vi "Teleop.vi"(10 "Match Info":T1={"Autonomous Elapsed Seconds"=0.0, "TeleOp Elapsed Seconds"=0.0, "Disabled Elapsed Seconds"=0.0, "Visited Autonomous"=FALSE, "Visited TeleOp"=FALSE, "Visited Disabled"=FALSE, "Autonomous Settings"={"Autonomous Style"=enum."Independent", "VI Refnum"=refnum}}, 11 "Call Context":T2) -> ()   [LabVIEW 2017]
doc: "This VI is called for each TeleOp packet received from the DS where the robot is not disabled. It is often used to read from the joysticks and update I/O or to update setpoints for timed control loops. It should complete and return within 20 milliseconds or it may miss DS packets."
uses:
  <vilib>/Rock Robotics/WPI/DriverStation/WPI_DriverStationDerivedRobotMode.ctl
  <vilib>/Rock Robotics/WPI/DriverStation/WPI_DriverStationMatch Info.ctl
  <vilib>/Rock Robotics/WPI/Solenoid/WPI_SolenoidValue.ctl
  <vilib>/Rock Robotics/WPI/Utilities/WPI_GetSetVariantRefNum.vi
  <vilib>/Rock Robotics/Network Tables/NT Read Boolean.vi
  <vilib>/Rock Robotics/Network Tables/NT Read Number.vi
  Robot Global Data.vi
  <vilib>/Rock Robotics/WPI/ThirdParty/Phoenix-LabVIEW/Motor Controller/Get/CTRE_Phoenix_MotorController_GetQuadratureData.vi
  <vilib>/Rock Robotics/WPI/Solenoid/WPI_SolenoidSetEnum.vi
panel:
  out "Sample Slider 0":dbl(slide) scale=0.0..5.0
  out "Sample Boolean 1":bool
  out "Sample Boolean 0":bool
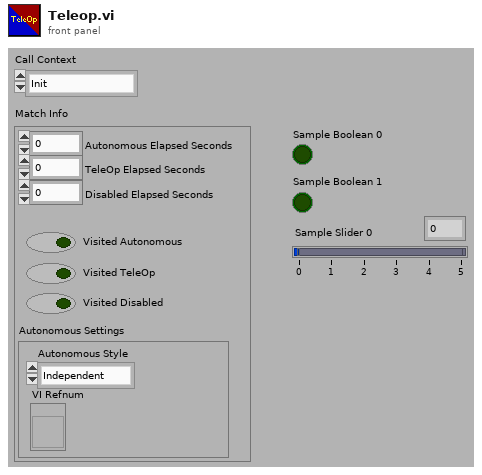
[diagram p1: front panel]
types:
  T1 = typedef "WPI_DriverStationMatch Info.ctl" = cluster{"Autonomous Elapsed Seconds":dbl, "TeleOp Elapsed Seconds":dbl, "Disabled Elapsed Seconds":dbl, "Visited Autonomous":bool, "Visited TeleOp":bool, "Visited Disabled":bool, "Autonomous Settings":cluster{"Autonomous Style":enum16{"Iterative", "Independent"}, "VI Refnum":refnum<vi>}}
  T2 = typedef "WPI_DriverStationDerivedRobotMode.ctl" = enum16{"Init", "Execute", "Stop"}
  T3 = typedef "WPI_SolenoidValue.ctl" = enum16{"Off", "On", "Forward", "Reverse"}
  T4 = typedef "WPI_JoystickDevRef.ctl" = cluster{"Device":T5}
  T5 = typedef "WPI_JoystickDeviceEnum.ctl" = enum16{"USB 0", "USB 1", "USB 2", "USB 3", "USB 4", "USB 5"}
  T6 = typedef "WPI_MotorControlDeviceRef.ctl" = cluster{"DeviceStatus":errorcluster, "Type":T7, "PWM":cluster{"PWM Channel":T8, "DeadBand":T9}, "CAN":cluster{"Device Number":u8, "SetOutput VI Ref":variant, "GetOutput VI Ref":variant, "Enable VI Ref":variant, "Disable VI Ref":variant, "Data":variant}, "Invert":bool, "DIO PWM":cluster{"PWM \"Enable\" Channel":T8, "DIOChannel":T10, "PWM Rate":dbl}}
  T7 = typedef "WPI_MotorControlType.ctl" = enum16{"PWM", "CAN", "DIO PWM"}
  T8 = typedef "FPGA_DIOPWMChannel.ctl" = enum8{"PWM 0", "PWM 1", "PWM 2", "PWM 3", "PWM 4", "PWM 5", "PWM 6", "PWM 7", "PWM 8", "PWM 9", "PWM MXP 0", "PWM MXP 1", "PWM MXP 2", "PWM MXP 3", "PWM MXP 4", "PWM MXP 5", "PWM MXP 6", "PWM MXP 7", "PWM MXP 8", "PWM MXP 9", "Invalid"}
  T9 = typedef "WPI_PWMDeadband.ctl" = cluster{"Name":string, "maxPositivePwm":i32, "minPositivePwm":i32, "centerPwm":i32, "maxNegativePwm":i32, "minNegativePwm":i32, "angularRange":u16}
  T10 = typedef "FPGA_DIOChannel.ctl" = enum8{"DIO 0", "DIO 1", "DIO 2", "DIO 3", "DIO 4", "DIO 5", "DIO 6", "DIO 7", "DIO 8", "DIO 9", "DIO MXP 0", "DIO MXP 1", "DIO MXP 2", "DIO MXP 3", "DIO MXP 4", "DIO MXP 5", "DIO MXP 6", "DIO MXP 7", "DIO MXP 8", "DIO MXP 9", "DIO MXP 10", "DIO MXP 11", "DIO MXP 12", "DIO MXP 13", "DIO MXP 14", "DIO MXP 15", "SPI Port CS1", "SPI Port CS2", "SPI Port CS3", "SPI Port MISO", "SPI Port MOSI", "Invalid"}
  T11 = typedef "WPI_SolenoidDevRef.ctl" = cluster{"DevStatus":errorcluster, "Pneumatics Control Module":u8, "Forward Solenoid Channel":T12, "Reverse Solenoid Channel":T12}
  T12 = typedef "WPI_SolenoidChannel.ctl" = enum8{"Solenoid 0", "Solenoid 1", "Solenoid 2", "Solenoid 3", "Solenoid 4", "Solenoid 5", "Solenoid 6", "Solenoid 7", "Invalid"}
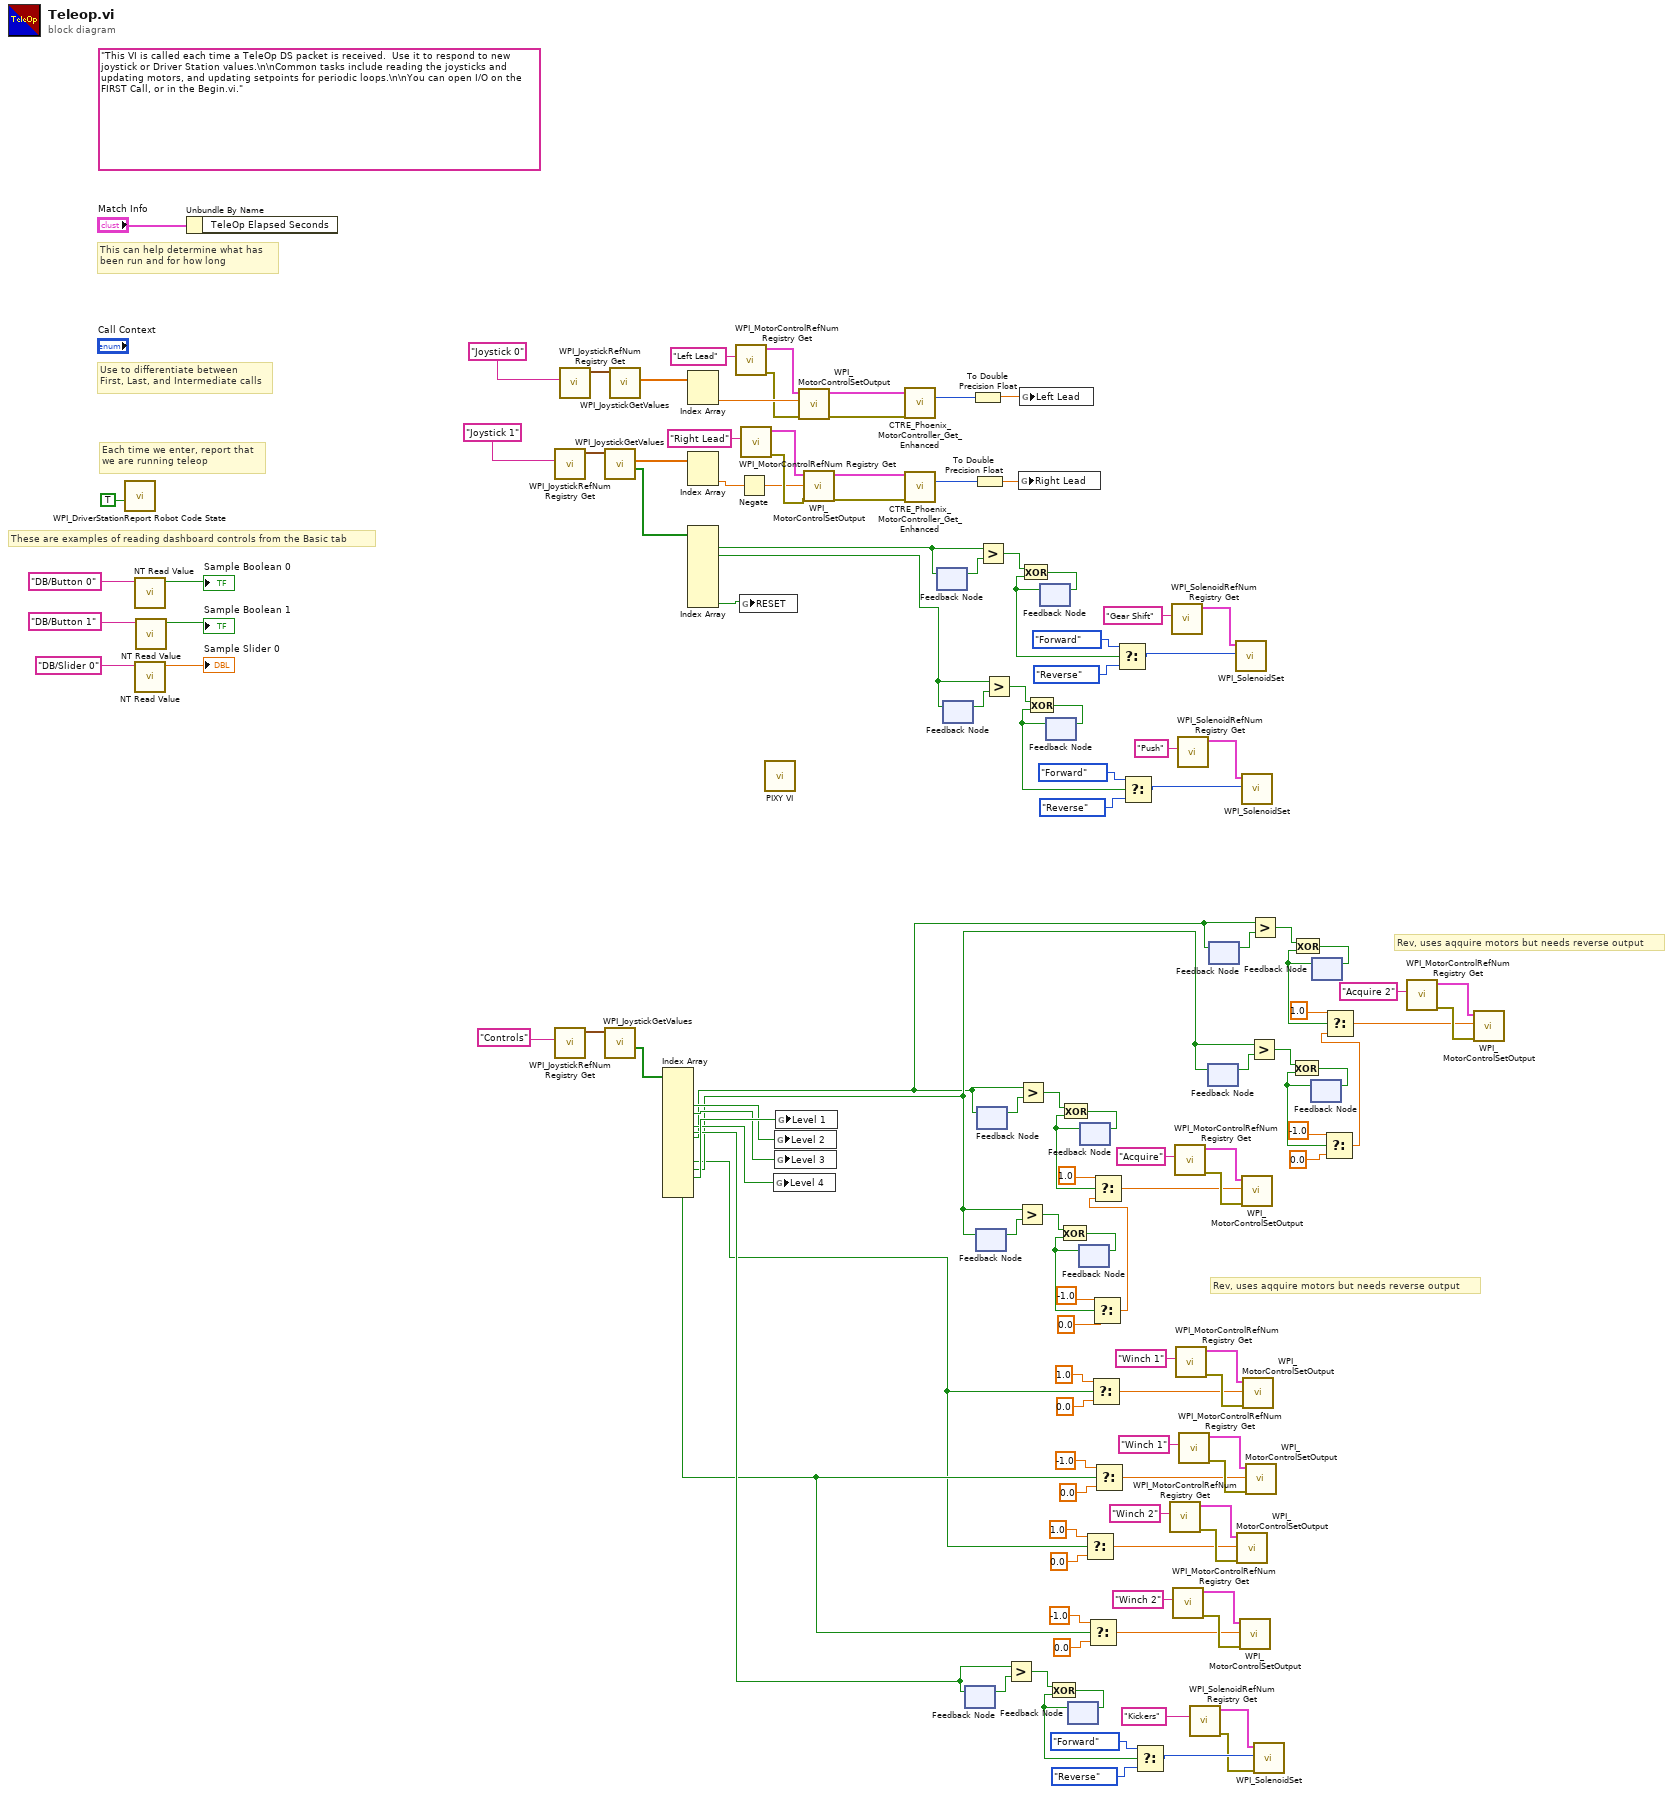
[diagram p0: block diagram]
diagram:
  (unwired) "This VI is called each time a TeleOp DS packet is received.  Use it to respond to new joystick or Driver Station values.\n\nCommon tasks include reading the joysticks and updating motors, and updating setpoints for periodic loops.\n\nYou can open I/O on the FIRST Call, or in the Begin.vi."
  # "Rev, uses aqquire motors but needs reverse output"
  # "Rev, uses aqquire motors but needs reverse output"
  # "These are examples of reading dashboard controls from the Basic tab"
  # "Each time we enter, report that\nwe are running teleop"
  # "Use to differentiate between\nFirst, Last, and Intermediate calls"
  # "This can help determine what has\nbeen run and for how long"
  n1 = call <vilib>:"WPI_DriverStationReport Robot Code State.vi"("TeleOp"=TRUE ("Autonomous")) -> ()  [unwired: 10 in, 1 out]
  n2 = call-poly <vilib>:"NT Read Value.vi"("Name"="DB/Button 0" ("refnum name")) -> ("Boolean"=→"Sample Boolean 0":bool)  [unwired: 9 in, 1 out]
  n3 = call-poly <vilib>:"NT Read Value.vi"("Name"="DB/Slider 0" ("refnum name")) -> ("Numeric"=→"Sample Slider 0":dbl)  [unwired: 9 in, 1 out]
  n4 = call-poly <vilib>:"NT Read Value.vi"("Name"="DB/Button 1" ("refnum name")) -> ("Boolean"=→"Sample Boolean 1":bool)  [unwired: 9 in, 1 out]
  n5 = Unbundle By Name("Match Info") -> ()  [unwired: 1 out]
  n6 = call <vilib>:"WPI_JoystickRefNum Registry Get.vi"("refnum name"="Joystick 1") -> ("JoystickDevRef"=w119:T4)  [unwired: 1 in, 9 out]
  n7 = call <vilib>:"WPI_JoystickRefNum Registry Get.vi"("refnum name"="Controls") -> ("JoystickDevRef"=w89:T4)  [unwired: 1 in, 9 out]
  n8 = call <vilib>:"WPI_JoystickRefNum Registry Get.vi"("refnum name"="Joystick 0") -> ("JoystickDevRef"=w129:T4)  [unwired: 1 in, 9 out]
  n9 = call <vilib>:"WPI_JoystickGetValues.vi"("JoystickDevRef"=w119) -> ("Buttons"=w112:bool[], "Axes"=w118:dbl[])  [unwired: 6 in, 3 out]
  n10 = call <vilib>:"WPI_JoystickGetValues.vi"("JoystickDevRef"=w89) -> ("Buttons"=w88:bool[])  [unwired: 6 in, 4 out]
  n11 = call <vilib>:"WPI_JoystickGetValues.vi"("JoystickDevRef"=w129) -> ("Axes"=w127:dbl[])  [unwired: 6 in, 4 out]
  n12 = Index Array(array=w88) -> (element #3=w36:bool, element #4=w38:bool, element #5=w37:bool, element #6=w35:bool, element #7=w16:bool, element #10=w1:bool, element #11=w17:bool, element #12=w39:bool, element #14=w2:bool)  [unwired: 14 in, 5 out]
  n13 = Index Array(array=w127) -> (element #1=w116:dbl)  [unwired: 2 in, 1 out]
  n14 = Index Array(array=w118) -> (element #2=w34:dbl)  [unwired: 2 in, 1 out]
  n15 = Index Array(array=w112) -> (element #1=w107:bool, element #2=w92:bool, element #8=w91:bool)  [unwired: 8 in, 5 out]
  n16 = call <vilib>:"WPI_MotorControlRefNum Registry Get.vi"("refnum name"="Left Lead") -> ("error out"=w78:errorcluster, "MotorControlDevRef"=w115:T6)  [unwired: 9 in]
  n17 = Negate(x=w34) -> (-x=w33:dbl)
  n18 = global write "Robot Global Data.vi" "RESET"(w91) -> ()
  n19 = call <vilib>:"WPI_MotorControlRefNum Registry Get.vi"("refnum name"="Right Lead") -> ("error out"=w79:errorcluster, "MotorControlDevRef"=w113:T6)  [unwired: 9 in]
  n20 = call "PIXY VI.vi"() -> ()  [unwired: 14 in, 6 out]
  n21 = global write "Robot Global Data.vi" "Level 4"(w37) -> ()
  n22 = global write "Robot Global Data.vi" "Level 2"(w36) -> ()
  n23 = global write "Robot Global Data.vi" "Level 3"(w38) -> ()
  n24 = global write "Robot Global Data.vi" "Level 1"(w39) -> ()
  n25 = call <vilib>:"WPI_MotorControlSetOutput.vi"("error in (no error)"=w78, "Output"=w116, "MotorControlDevRef"=w115) -> ("error out"=w63:errorcluster, "MotorControlDevRef"=w64:T6)  [unwired: 6 in, 1 out]
  n26 = call <vilib>:"WPI_MotorControlSetOutput.vi"("error in (no error)"=w79, "Output"=w33, "MotorControlDevRef"=w113) -> ("error out"=w59:errorcluster, "MotorControlDevRef"=w60:T6)  [unwired: 6 in, 1 out]
  n27 = call-poly <vilib>:"CTRE_Phoenix_MotorController_Get_Enhanced.vi"("PhoenixMotorControlDevRef"=w64, "error in"=w63) -> ("Quadrature Position"=w62:i32)  [unwired: 10 in, 3 out]
  n28 = call-poly <vilib>:"CTRE_Phoenix_MotorController_Get_Enhanced.vi"("PhoenixMotorControlDevRef"=w60, "error in"=w59) -> ("Quadrature Position"=w61:i32)  [unwired: 10 in, 3 out]
  n29 = feedback #1() -> (w108:bool)  [unwired: 1 in]
  n30 = feedback-in #1(w107) -> ()
  n31 = feedback #2() -> (w98:bool)  [unwired: 1 in]
  n32 = feedback-in #2(w92) -> ()
  n33 = feedback #3() -> (w45:bool)  [unwired: 1 in]
  n34 = feedback-in #3(w35) -> ()
  n35 = To Double Precision Float(number=w62) -> (double precision float=w58:dbl)
  n36 = To Double Precision Float(number=w61) -> (double precision float=w57:dbl)
  n37 = feedback #4() -> (w75:bool)  [unwired: 1 in]
  n38 = feedback-in #4(w17) -> ()
  n39 = feedback #5() -> (w85:bool)  [unwired: 1 in]
  n40 = feedback-in #5(w16) -> ()
  n41 = Greater?(x=w107, y=w108) -> (0:w111:bool)
  n42 = Greater?(x=w92, y=w98) -> (0:w101:bool)
  n43 = Greater?(x=w35, y=w45) -> (0:w46:bool)
  n44 = Greater?(x=w17, y=w75) -> (0:w77:bool)
  n45 = Greater?(x=w16, y=w85) -> (0:w87:bool)
  n46 = global write "Robot Global Data.vi" "Right Lead"(w57) -> ()
  n47 = global write "Robot Global Data.vi" "Left Lead"(w58) -> ()
  n48 = feedback #6() -> (w109:bool)  [unwired: 1 in]
  n49 = Exclusive Or(1:w109, 2:w111) -> (0:w110:bool)
  n50 = feedback-in #6(w110) -> ()
  n51 = feedback #7() -> (w99:bool)  [unwired: 1 in]
  n52 = Exclusive Or(1:w99, 2:w101) -> (0:w100:bool)
  n53 = feedback-in #7(w100) -> ()
  n54 = feedback #8() -> (w43:bool)  [unwired: 1 in]
  n55 = Exclusive Or(1:w43, 2:w46) -> (0:w44:bool)
  n56 = feedback-in #8(w44) -> ()
  n57 = feedback #9() -> (w74:bool)  [unwired: 1 in]
  n58 = Exclusive Or(1:w74, 2:w77) -> (0:w76:bool)
  n59 = feedback-in #9(w76) -> ()
  n60 = feedback #10() -> (w84:bool)  [unwired: 1 in]
  n61 = Exclusive Or(1:w84, 2:w87) -> (0:w86:bool)
  n62 = feedback-in #10(w86) -> ()
  n63 = Select(t=1.0, s=w1, f=0.0) -> (s? t:f=w9:dbl)
  n64 = Select(t=-1.0, s=w2, f=0.0) -> (s? t:f=w5:dbl)
  n65 = Select(t=1.0, s=w1, f=0.0) -> (s? t:f=w66:dbl)
  n66 = Select(t=-1.0, s=w74, f=0.0) -> (s? t:f=w42:dbl)
  n67 = Select(t=1.0, s=w84, f=w42) -> (s? t:f=w65:dbl)
  n68 = Select(t=-1.0, s=w2, f=0.0) -> (s? t:f=w53:dbl)
  n69 = Select(t=WPI_SolenoidValue."Forward" ("Value"), s=w109, f=WPI_SolenoidValue."Reverse" ("Value")) -> (s? t:f=w102:T3)
  n70 = Select(t=WPI_SolenoidValue."Forward" ("Value"), s=w99, f=WPI_SolenoidValue."Reverse" ("Value")) -> (s? t:f=w93:T3)
  n71 = Select(t=WPI_SolenoidValue."Forward" ("Value"), s=w43, f=WPI_SolenoidValue."Reverse" ("Value")) -> (s? t:f=w49:T3)
  n72 = call <vilib>:"WPI_MotorControlRefNum Registry Get.vi"("refnum name"="Winch 2") -> ("error out"=w10:errorcluster, "MotorControlDevRef"=w11:T6)  [unwired: 9 in]
  n73 = call <vilib>:"WPI_SolenoidRefNum Registry Get.vi"("refnum name"="Gear Shift") -> ("SolenoidDevRef"=w105:T11)  [unwired: 9 in, 1 out]
  n74 = call <vilib>:"WPI_MotorControlRefNum Registry Get.vi"("refnum name"="Winch 2") -> ("error out"=w6:errorcluster, "MotorControlDevRef"=w4:T6)  [unwired: 9 in]
  n75 = call <vilib>:"WPI_MotorControlRefNum Registry Get.vi"("refnum name"="Acquire") -> ("error out"=w80:errorcluster, "MotorControlDevRef"=w81:T6)  [unwired: 9 in]
  n76 = call <vilib>:"WPI_MotorControlRefNum Registry Get.vi"("refnum name"="Winch 1") -> ("error out"=w67:errorcluster, "MotorControlDevRef"=w68:T6)  [unwired: 9 in]
  n77 = call <vilib>:"WPI_SolenoidRefNum Registry Get.vi"("refnum name"="Push") -> ("SolenoidDevRef"=w96:T11)  [unwired: 9 in, 1 out]
  n78 = call <vilib>:"WPI_MotorControlRefNum Registry Get.vi"("refnum name"="Winch 1") -> ("error out"=w54:errorcluster, "MotorControlDevRef"=w52:T6)  [unwired: 9 in]
  n79 = call <vilib>:"WPI_SolenoidRefNum Registry Get.vi"("refnum name"="Kickers") -> ("error out"=w47:errorcluster, "SolenoidDevRef"=w48:T11)  [unwired: 9 in]
  n80 = feedback #11() -> (w22:bool)  [unwired: 1 in]
  n81 = feedback-in #11(w17) -> ()
  n82 = feedback #12() -> (w30:bool)  [unwired: 1 in]
  n83 = feedback-in #12(w16) -> ()
  n84 = call-poly <vilib>:"WPI_SolenoidSet.vi"("Value"=w102, "SolenoidDevRef"=w105) -> ()  [unwired: 8 in, 2 out]
  n85 = call <vilib>:"WPI_MotorControlSetOutput.vi"("error in (no error)"=w10, "Output"=w9, "MotorControlDevRef"=w11) -> ()  [unwired: 6 in, 3 out]
  n86 = call <vilib>:"WPI_MotorControlSetOutput.vi"("error in (no error)"=w6, "Output"=w5, "MotorControlDevRef"=w4) -> ()  [unwired: 6 in, 3 out]
  n87 = call-poly <vilib>:"WPI_SolenoidSet.vi"("Value"=w93, "SolenoidDevRef"=w96) -> ()  [unwired: 8 in, 2 out]
  n88 = call <vilib>:"WPI_MotorControlSetOutput.vi"("error in (no error)"=w80, "Output"=w65, "MotorControlDevRef"=w81) -> ()  [unwired: 6 in, 3 out]
  n89 = call <vilib>:"WPI_MotorControlSetOutput.vi"("error in (no error)"=w67, "Output"=w66, "MotorControlDevRef"=w68) -> ()  [unwired: 6 in, 3 out]
  n90 = call <vilib>:"WPI_MotorControlSetOutput.vi"("error in (no error)"=w54, "Output"=w53, "MotorControlDevRef"=w52) -> ()  [unwired: 6 in, 3 out]
  n91 = Greater?(x=w17, y=w22) -> (0:w24:bool)
  n92 = Greater?(x=w16, y=w30) -> (0:w32:bool)
  n93 = call-poly <vilib>:"WPI_SolenoidSet.vi"("error in (no error)"=w47, "Value"=w49, "SolenoidDevRef"=w48) -> ()  [unwired: 7 in, 2 out]
  n94 = feedback #13() -> (w21:bool)  [unwired: 1 in]
  n95 = Exclusive Or(1:w21, 2:w24) -> (0:w23:bool)
  n96 = feedback-in #13(w23) -> ()
  n97 = feedback #14() -> (w29:bool)  [unwired: 1 in]
  n98 = Exclusive Or(1:w29, 2:w32) -> (0:w31:bool)
  n99 = feedback-in #14(w31) -> ()
  n100 = Select(t=-1.0, s=w21, f=0.0) -> (s? t:f=w18:dbl)
  n101 = Select(t=1.0, s=w29, f=w18) -> (s? t:f=w19:dbl)
  n102 = call <vilib>:"WPI_MotorControlRefNum Registry Get.vi"("refnum name"="Acquire 2") -> ("error out"=w25:errorcluster, "MotorControlDevRef"=w26:T6)  [unwired: 9 in]
  n103 = call <vilib>:"WPI_MotorControlSetOutput.vi"("error in (no error)"=w25, "Output"=w19, "MotorControlDevRef"=w26) -> ()  [unwired: 6 in, 3 out]
